vi "LIDAR Position from Inertial Position.vi"(10 "CM X, Y, Theta":dbl[](array[numeric])=[0.0, 0.0, 0.0]) -> (2 "LIDAR X, Y, Theta":dbl[](array[numeric]))   [LabVIEW 2012]
uses:
  Robot Parameters.vi
  <vilib>/Analysis/coordinate.llb/2D Cartesian Coordinate Rotation (Scalar).vi
  <vilib>/Analysis/NI_AALPro.lvlib
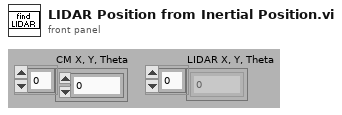
[diagram p1: front panel]
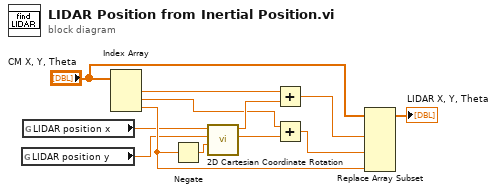
[diagram p0: block diagram]
diagram:
  n1 = global read "Robot Parameters.vi" "LIDAR position y"() -> (w1:dbl)
  n2 = global read "Robot Parameters.vi" "LIDAR position x"() -> (w2:dbl)
  n3 = Index Array(array="CM X, Y, Theta") -> (element #1=w8:dbl, element #2=w6:dbl, element #3=w9:dbl)  [unwired: 3 in]
  n4 = Negate(x=w9) -> (-x=w10:dbl)
  n5 = call-poly <vilib>:"2D Cartesian Coordinate Rotation.vi"("theta"=w10, "y"=w1, "x"=w2) -> ("y out"=w5:dbl, "x out"=w7:dbl)  [unwired: 6 in, 1 out]
  n6 = Add(x=w8, y=w7) -> (x+y=w4:dbl)
  n7 = Add(x=w6, y=w5) -> (x+y=w3:dbl)
  n8 = Replace Array Subset(array="CM X, Y, Theta", new element #1=w4, new element #2=w3, new element #3=w9) -> (→"LIDAR X, Y, Theta":dbl[])  [unwired: 3 in]
